vi "GEA3 HexStringToU64.vi"(0 "Input String":string, 7 "Starting Offset":i32) -> (4 "Number Out":u64)   [LabVIEW 2016]
doc: "Takes an input from \"String Input\" in the form of a 32-bit integer with spaces between bytes starting at \"Starting Offset\" and converts it to a U32 integer output, \"Number Out.\""
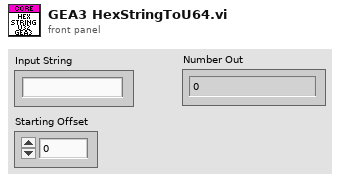
[diagram p1: front panel]
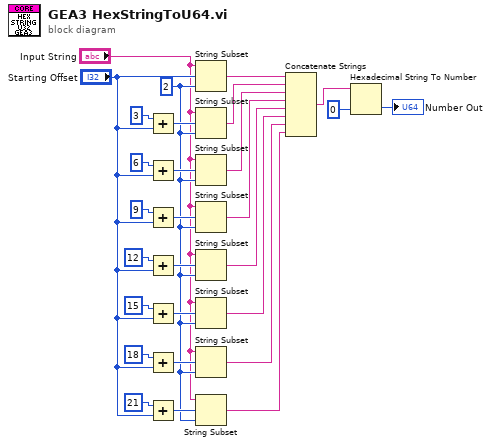
[diagram p0: block diagram]
diagram:
  w5 = 2 ("offset (0)")
  n1 = Add(x=3, y="Starting Offset") -> (x+y=w22:i32)
  n2 = Add(x=6, y="Starting Offset") -> (x+y=w19:i32)
  n3 = Add(x=9, y="Starting Offset") -> (x+y=w18:i32)
  n4 = Add(x=12, y="Starting Offset") -> (x+y=w14:i32)
  n5 = Add(x=15, y="Starting Offset") -> (x+y=w11:i32)
  n6 = Add(x=18, y="Starting Offset") -> (x+y=w8:i32)
  n7 = Add(x=21, y="Starting Offset") -> (x+y=w6:i32)
  n8 = String Subset(string="Input String", offset (0)="Starting Offset", length (rest)=w5) -> (substring=w26:string)
  n9 = String Subset(string="Input String", offset (0)=w22, length (rest)=w5) -> (substring=w25:string)
  n10 = String Subset(string="Input String", offset (0)=w19, length (rest)=w5) -> (substring=w17:string)
  n11 = String Subset(string="Input String", offset (0)=w18, length (rest)=w5) -> (substring=w16:string)
  n12 = String Subset(string="Input String", offset (0)=w14, length (rest)=w5) -> (substring=w13:string)
  n13 = String Subset(string="Input String", offset (0)=w11, length (rest)=w5) -> (substring=w10:string)
  n14 = String Subset(string="Input String", offset (0)=w8, length (rest)=w5) -> (substring=w3:string)
  n15 = String Subset(string="Input String", offset (0)=w6, length (rest)=w5) -> (substring=w2:string)
  n16 = Concatenate Strings(w26, w25, w17, w16, w13, w10, w3, w2) -> (w28:string)
  n17 = Hexadecimal String To Number(string=w28, default (0uL)=u64 0) -> (number=→"Number Out":u64)  [unwired: 1 in, 1 out]
